vi "PH_IEEE1394Camera.set Ring Cam Attribute Tip Strip.vi"(2 "EnumValues[]":u32[](array[numeric]), 3 "EnumStrings[]":string[](array[string]), 4 "Attribute Name":string) -> (0 "Strings and Values":cluster{"String":string, "Value":u32}[](array[cluster]), 1 "Tip Strip":string)   [LabVIEW 2014, in "PH_IEEE1394Camera.lvlib"]
uses:
  PH_IEEE1394Camera.lvlib
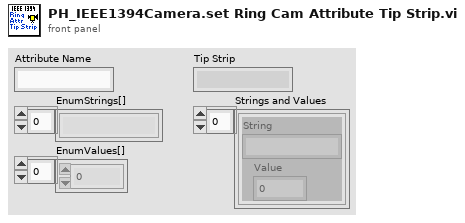
[diagram p1: front panel]
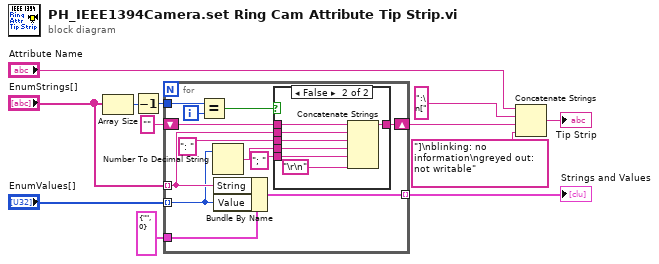
[diagram p0: block diagram]
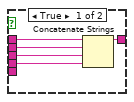
[diagram p2: hidden frame]
diagram:
  n1 = Array Size(array="EnumStrings[]") -> (size(s)=w9:i32)
  n2 = Decrement(x=w9) -> (x-1=w10:i32)
  n3 = for {
    tunnel: cluster{"String":string, "Value":u32} {"String"="", "Value"=0} -> [w13]
    tunnel: [w24] -> w12 mode=indexing
    tunnel: "EnumStrings[]" -> [w23] mode=indexing
    tunnel: "EnumValues[]" -> [w21] mode=indexing
    shift-right: [w18] -> w5
    shift-left: "" -> [w17]
    tunnel: w10 -> [w16]
    i -> [w15]
    n4 = Equal?(x=w16, y=w15) -> (x = y?=w14:bool)
    n5 = Number To Decimal String(number=w21) -> (decimal integer string=w20:string)  [unwired: 1 in]
    n6 = Bundle By Name(cluster=w13, "String"=w23, "Value"=w21) -> (w24:cluster{"String":string, "Value":u32})
    n7 = case shown="False" w14 {
      tunnel: w23 -> [w29 w36]
      tunnel: ": " ("string") -> [w28 w35]
      tunnel: w20 -> [w27 w34]
      tunnel: "; " ("string") -> [_ w33]
      tunnel: [w26 w32] -> w18
      tunnel: w17 -> [w25 w31]
      frame True {
        n8 = Concatenate Strings(w25, w29, w28, w27) -> (w26:string)
      }
      frame False {
        n9 = Concatenate Strings(w31, w36, w35, w34, w33, "\r\n") -> (w32:string)
      }
    }
  }
  "Strings and Values" <- w12
  n10 = Concatenate Strings("Attribute Name", ":\n[" ("string"), w5, "]\nblinking: no information\ngreyed out: not writable") -> (→"Tip Strip":string)
